vi "MorseCodeForLoop.vi"() -> ()   [LabVIEW 2020]
panel:
  out "MorseOutput":string
  in  "English input":string
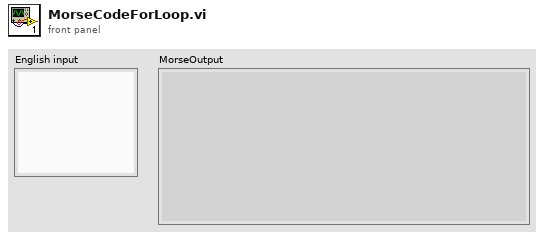
[diagram p1: front panel]
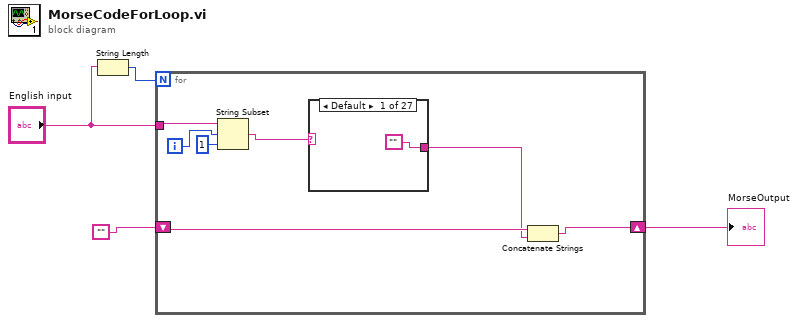
[diagram p0: block diagram]
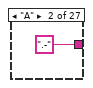
[diagram p2: hidden frame]
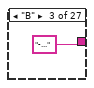
[diagram p3: hidden frame]
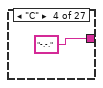
[diagram p4: hidden frame]
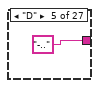
[diagram p5: hidden frame]
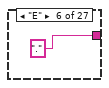
[diagram p6: hidden frame]
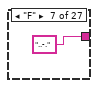
[diagram p7: hidden frame]
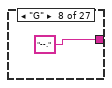
[diagram p8: hidden frame]
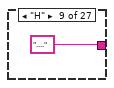
[diagram p9: hidden frame]
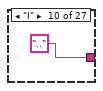
[diagram p10: hidden frame]
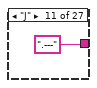
[diagram p11: hidden frame]
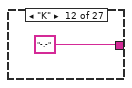
[diagram p12: hidden frame]
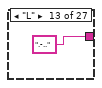
[diagram p13: hidden frame]
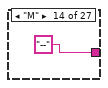
[diagram p14: hidden frame]
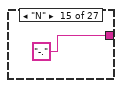
[diagram p15: hidden frame]
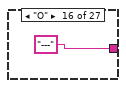
[diagram p16: hidden frame]
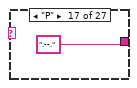
[diagram p17: hidden frame]
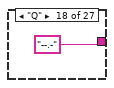
[diagram p18: hidden frame]
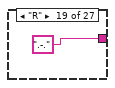
[diagram p19: hidden frame]
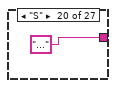
[diagram p20: hidden frame]
diagram:
  n1 = String Length(string="English input") -> (length=w1:i32)
  n2 = for {
    N: w1 -> [_]
    shift-right: [w7] -> w3
    shift-left: "" -> [w6]
    tunnel: "English input" -> [w11]
    i -> [w9]
    n3 = String Subset(string=w11, offset (0)=w9, length (rest)=1 ("length (rest)")) -> (substring=w8:string)
    n4 = case shown="Default" w8 {
      tunnel: ["" ".-" "-..." "-.-." "-.." "." "..-." "--." "...." ".." ".---" "-.-" ".-.." "--" "-." "---" ".--." "--.-" ".-." "..." "-" "..-" "...-" ".--" "-..-" "-.--" "--.."] -> w5
      frame Default {
      }
      frame "A" {
      }
      frame "B" {
      }
      frame "C" {
      }
      frame "D" {
      }
      frame "E" {
      }
      frame "F" {
      }
      frame "G" {
      }
      frame "H" {
      }
      frame "I" {
      }
      frame "J" {
      }
      frame "K" {
      }
      frame "L" {
      }
      frame "M" {
      }
      frame "N" {
      }
      frame "O" {
      }
      frame "P" {
      }
      frame "Q" {
      }
      frame "R" {
      }
      frame "S" {
      }
      frame "T" {
      }
      frame "U" {
      }
      frame "V" {
      }
      frame "W" {
      }
      frame "X" {
      }
      frame "Y" {
      }
      frame "Z" {
      }
    }
    n5 = Concatenate Strings(w6, w5) -> (w7:string)
  }
  "MorseOutput" <- w3
